vi "test Read U64 Array.vi"(8 "error in (no error)":errorcluster, 11 "TestCase in":refnum<class "Buffer Tests.lvclass">) -> (0 "error out":errorcluster, 3 "TestCase out":refnum<class "Buffer Tests.lvclass">)   [LabVIEW 2017, in "Buffer Tests.lvclass"]
uses:
  Buffer Tests.lvclass
  Classes/Buffer/Buffer.lvclass
  C:/Git/DSF/LabVIEW-Memory/Source/Classes/Pointer/Pointer.lvclass
  Classes/Buffer/Read Buffer 1D U64.vi
  <vilib>/addons/_JKI Toolkits/VI Tester/TestCase.llb/TestCase.lvclass
  LabVIEW-Memory/Source/Classes/Pointer/Pointer.lvclass
  C:/Program Files (x86)/National Instruments/LabVIEW 2017/vi.lib/addons/_JKI Toolkits/VI Tester/TestCase.llb/TestCase.lvclass
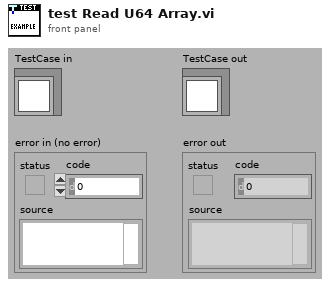
[diagram p1: front panel]
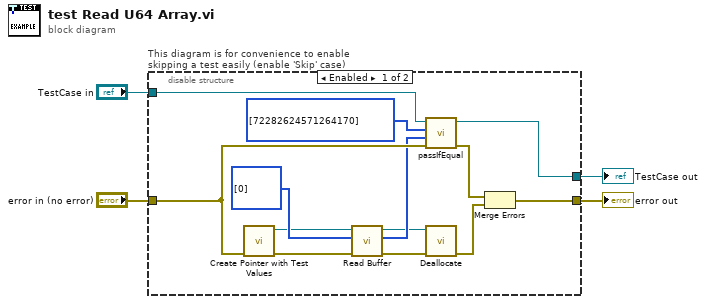
[diagram p0: block diagram]
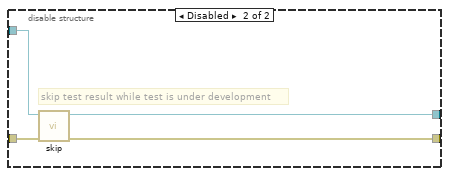
[diagram p2: hidden frame]
diagram:
  n1 = disable-structure "This diagram is for convenience to enable skipping a test easily (enable 'Skip' case)" shown="Enabled" {
    disable-tunnel: "TestCase in" -> [w15 w21]
    disable-tunnel: [w16 w19] -> w1
    disable-tunnel: [w13 w20] -> w2
    disable-tunnel: "error in (no error)" -> [w14 w18]
    frame Enabled {
      n2 = call "Create Pointer with Test Values.vi"("error in (no error)"=w14) -> ("error out"=w8:errorcluster, "Buffer out"=w7:refnum<class "Buffer.lvclass">)  [unwired: 9 in]
      n3 = call-poly "Read Buffer.vi"("error in (no error)"=w8, "dst array in"=u64[] [0] ("buffer in"), "Buffer in"=w7) -> ("error out"=w12:errorcluster, "dst array out"=w9:u64[], "Buffer out"=w5:refnum<class "Buffer.lvclass">)  [unwired: 5 in, 1 out]
      n4 = call-dynamic "passIfEqual.vi"("error in (no error)"=w14, "y"=w9, "x"=u64[] [72282624571264170] ("reversed array 4"), "TestCase in"=w15) -> ("error out"=w17:errorcluster, "TestCase out"=w16:refnum<class "Buffer Tests.lvclass">)  [unwired: 6 in]
      n5 = call "Deallocate.vi"("error in (no error)"=w12, "Pointer in"=w5) -> ("error out"=w6:errorcluster)  [unwired: 8 in, 1 out]
      n6 = Merge Errors(w17, w6) -> (w13:errorcluster)
    }
    frame Disabled {
      # "skip test result while test is under development"
      n7 = call <vilib>:"skip.vi"("error in (no error)"=w18, "TestCase in"=w21) -> ("error out"=w20:errorcluster, "TestCase out"=w19:refnum<class "Buffer Tests.lvclass">)  [unwired: 8 in]
    }
  }
  "error out" <- w2
  "TestCase out" <- w1
